vi "Formula_KG.vi"(6 "KTu":dbl[](array[numeric]), 7 "Tripped Time":i32[](array[numeric]), 8 "error in":errorcluster, 9 "consTime":i32, 10 "Load Time":i32, 11 "Preload Time":i32) -> (0 "error out":errorcluster, 3 "KGR":dbl[](array[numeric]))   [LabVIEW 2015]
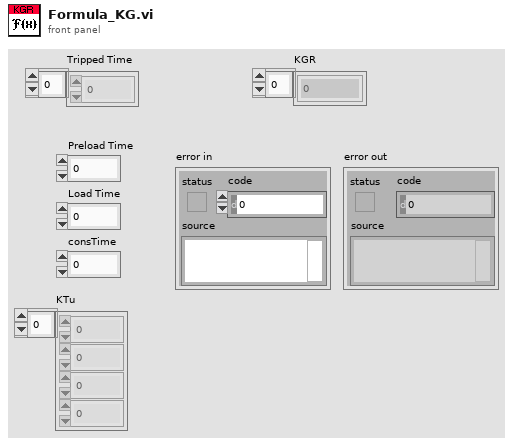
[diagram p1: front panel]
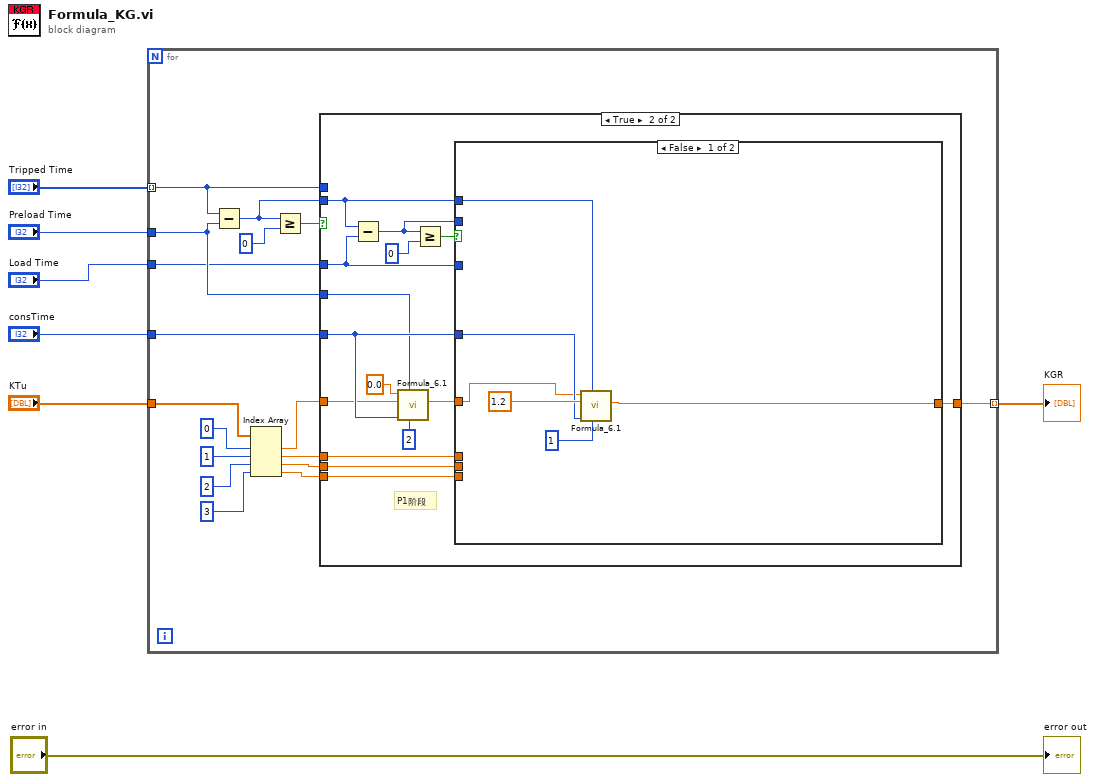
[diagram p0: block diagram]
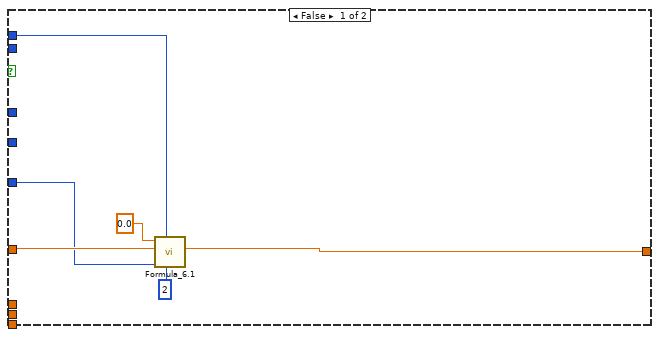
[diagram p2: hidden frame]
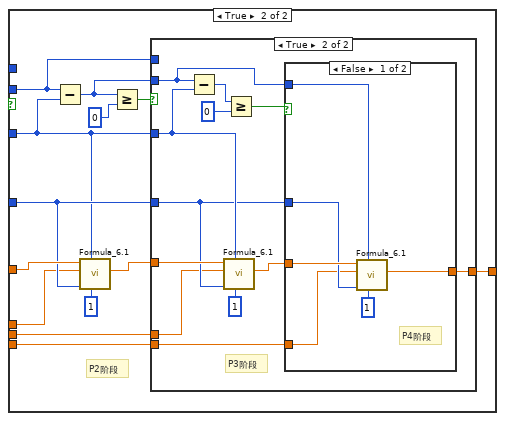
[diagram p3: hidden frame]
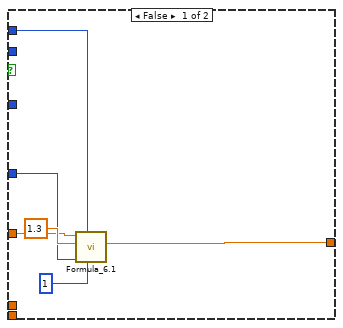
[diagram p4: hidden frame]
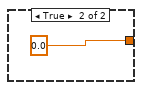
[diagram p5: hidden frame]
diagram:
  n1 = for {
    tunnel: "Tripped Time" -> [w8] mode=indexing
    tunnel: [w24] -> w2 mode=indexing
    tunnel: "KTu" -> [w23]
    tunnel: "Preload Time" -> [w22]
    tunnel: "Load Time" -> [w21]
    tunnel: "consTime" -> [w20]
    n2 = Subtract(x=w8, y=w22) -> (x-y=w17:i32)
    n3 = Index Array(array=w23, index #1=0 ("index"), index #2=1 ("index"), index #3=2 ("index"), index #4=3 ("index")) -> (element #1=w12:dbl, element #2=w11:dbl, element #3=w10:dbl, element #4=w9:dbl)
    n4 = Greater Or Equal?(x=w17, y=0) -> (x >= y?=w18:bool)
    n5 = case shown="True" w18 {
      tunnel: w20 -> [w27 w41]
      tunnel: w22 -> [_ w40]
      tunnel: w17 -> [_ w36]
      tunnel: w21 -> [_ w39]
      tunnel: [w26 w38] -> w24
      tunnel: w12 -> [w29 w34]
      tunnel: w11 -> [_ w33]
      tunnel: w10 -> [_ w32]
      tunnel: w9 -> [_ w31]
      tunnel: w8 -> [w25 _]
      frame False {
        n6 = call "Formula_6.1.vi"("x"=2, "t_aus"=w25, "t"=w27, "K_last"=w29, "K_vor"=0.0) -> ("K_Gr"=w26:dbl)  [unwired: 6 in]
      }
      frame True {
        # "P1阶段"
        n7 = Subtract(x=w36, y=w39) -> (x-y=w37:i32)
        n8 = call "Formula_6.1.vi"("x"=2, "t_aus"=w40, "t"=w41, "K_last"=w34, "K_vor"=0.0) -> ("K_Gr"=w42:dbl)  [unwired: 6 in]
        n9 = Greater Or Equal?(x=w37, y=0) -> (x >= y?=w43:bool)
        n10 = case shown="False" w43 {
          tunnel: w42 -> [w49 w64]
          tunnel: w41 -> [w50 w61]
          tunnel: w37 -> [_ w52]
          tunnel: w39 -> [_ w59]
          tunnel: [w48 w58] -> w38
          tunnel: w36 -> [w47 _]
          tunnel: w33 -> [_ w55]
          tunnel: w32 -> [_ w54]
          tunnel: w31 -> [_ w53]
          frame False {
            n11 = call "Formula_6.1.vi"("x"=1, "t_aus"=w47, "t"=w50, "K_last"=1.2, "K_vor"=w49) -> ("K_Gr"=w48:dbl)  [unwired: 6 in]
          }
          frame True {
            # "P2阶段"
            n12 = Subtract(x=w52, y=w59) -> (x-y=w57:i32)
            n13 = call "Formula_6.1.vi"("x"=1, "t_aus"=w59, "t"=w61, "K_last"=w55, "K_vor"=w64) -> ("K_Gr"=w60:dbl)  [unwired: 6 in]
            n14 = Greater Or Equal?(x=w57, y=0) -> (x >= y?=w62:bool)
            n15 = case shown="True" w62 {
              tunnel: w61 -> [w69 w78]
              tunnel: w60 -> [w68 w82]
              tunnel: w57 -> [_ w74]
              tunnel: w59 -> [_ w80]
              tunnel: [w67 w75] -> w58
              tunnel: w52 -> [w66 _]
              tunnel: w54 -> [_ w72]
              tunnel: w53 -> [_ w71]
              frame False {
                n16 = call "Formula_6.1.vi"("x"=1, "t_aus"=w66, "t"=w69, "K_last"=1.3, "K_vor"=w68) -> ("K_Gr"=w67:dbl)  [unwired: 6 in]
              }
              frame True {
                # "P3阶段"
                n17 = Subtract(x=w74, y=w80) -> (x-y=w76:i32)
                n18 = call "Formula_6.1.vi"("x"=1, "t_aus"=w80, "t"=w78, "K_last"=w72, "K_vor"=w82) -> ("K_Gr"=w77:dbl)  [unwired: 6 in]
                n19 = Greater Or Equal?(x=w76, y=0) -> (x >= y?=w79:bool)
                n20 = case shown="False" w79 {
                  tunnel: w78 -> [w87 _]
                  tunnel: w77 -> [w88 _]
                  tunnel: w74 -> [w86 _]
                  tunnel: [w84 0.0 ("K_last")] -> w75
                  tunnel: w71 -> [w83 _]
                  frame False {
                    # "P4阶段"
                    n21 = call "Formula_6.1.vi"("x"=1, "t_aus"=w86, "t"=w87, "K_last"=w83, "K_vor"=w88) -> ("K_Gr"=w84:dbl)  [unwired: 6 in]
                  }
                  frame True {
                  }
                }
              }
            }
          }
        }
      }
    }
  }
  "KGR" <- w2
  "error out" <- "error in"
